vi "Get All LogMeasData from Q.vi"(8 "error in (no error)":errorcluster) -> (0 "error out":errorcluster, 1 "MeasData[] out":T1[](array[typedef]), 2 "NumElements":i32, 3 "orData out":T4)   [LabVIEW 2019]
doc: "Developed by Kevin Thompson\nThompson Engineering, LLC\nkevin@thompsonengineering.net"
uses:
  TD MeasData--cluster.ctl
  TD MeasData QRef.ctl
  GBL DataQ Ref.vi
  DataTypes/InverterData--cluster.ctl
  DataTypes/InverterPhaseData--cluster.ctl
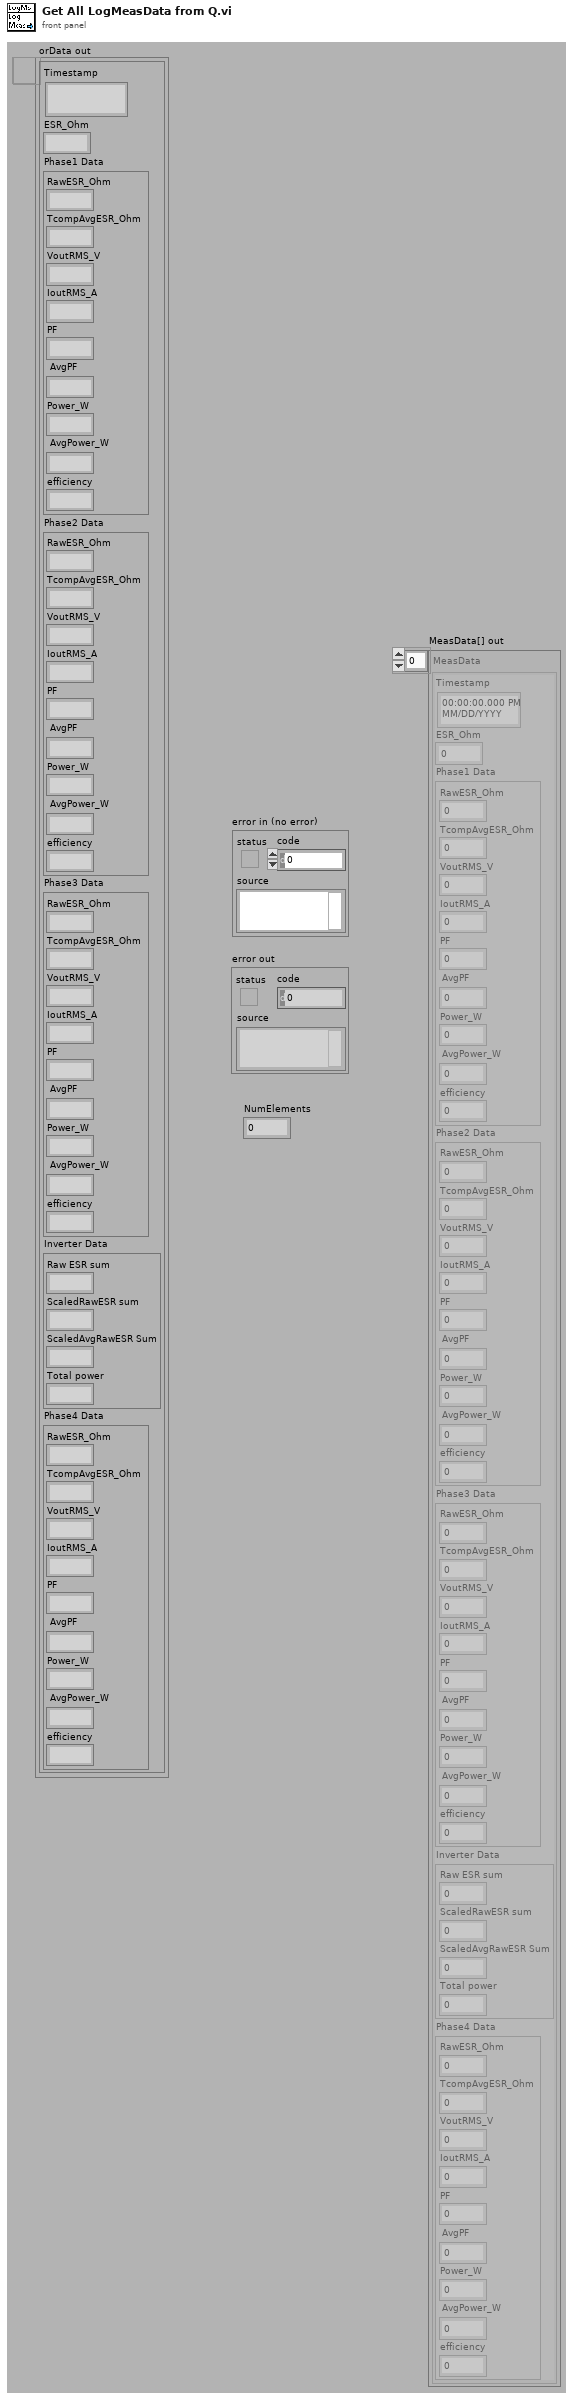
[diagram p1: front panel]
types:
  T1 = typedef "TD MeasData--cluster.ctl" = cluster{"Timestamp":timestamp, "ESR_Ohm":dbl, "Phase1 Data":T2, "Phase2 Data":T2, "Phase3 Data":T2, "Inverter Data":T3, "Phase4 Data":T2}
  T2 = typedef "InverterPhaseData--cluster.ctl" = cluster{"RawESR_Ohm":dbl, "TcompAvgESR_Ohm":dbl, "VoutRMS_V":dbl, "IoutRMS_A":dbl, "PF":dbl, "AvgPF":dbl, "Power_W":dbl, "AvgPower_W":dbl, "efficiency":dbl}
  T3 = typedef "InverterData--cluster.ctl" = cluster{"Raw ESR sum":dbl, "ScaledRawESR sum":dbl, "ScaledAvgRawESR Sum":dbl, "Total power":dbl}
  T4 = typedef "TD MeasData QRef.ctl" = refnum<queue>
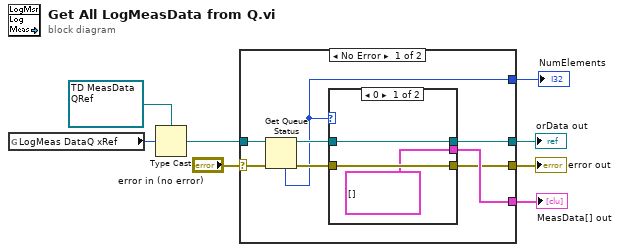
[diagram p0: block diagram]
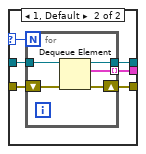
[diagram p2: hidden frame]
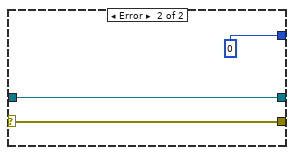
[diagram p3: hidden frame]
diagram:
  n1 = global read "GBL DataQ Ref.vi" "LogMeas DataQ xRef"() -> (w1:u32)
  n2 = Type Cast(type=T4 refnum ("orData out"), x=w1) -> (*(type *) &x=w5:T4)
  n3 = case shown="No Error" "error in (no error)" {
    selector: "error in (no error)" -> [w16 w32]
    tunnel: w5 -> [w15 w33]
    tunnel: [w10 w32] -> w8
    tunnel: [w14 w33] -> w7
    tunnel: [w11 _] -> w4
    tunnel: [w9 0 ("# elements in queue")] -> w3
    frame No Error {
      n4 = Get Queue Status(queue=w15, error in (no error)=w16) -> (queue out=w13:T4, error out=w12:errorcluster, # elements in queue=w9:i32)  [unwired: 1 in, 5 out]
      n5 = case shown="0" w9 {
        selector: w9 -> [_ w20]
        tunnel: [w19 w25] -> w14
        tunnel: w13 -> [w19 w24]
        tunnel: w12 -> [w18 w23]
        tunnel: [T1[] [] ("MeasData[] out") w22] -> w11
        tunnel: [w18 w21] -> w10
        frame 0 {
        }
        frame 1, Default {
          n6 = for {
            N: w20 -> [_]
            tunnel: [w30] -> w22 mode=indexing
            tunnel: [w29] -> w25
            tunnel: w24 -> [w28]
            shift-right: [w27] -> w21
            shift-left: w23 -> [w26]
            n7 = Dequeue Element(queue=w28, error in (no error)=w26) -> (queue out=w29:T4, element=w30:T1, error out=w27:errorcluster)  [unwired: 1 in, 1 out]
          }
        }
      }
    }
    frame Error {
    }
  }
  "orData out" <- w7
  "error out" <- w8
  "MeasData[] out" <- w4
  "NumElements" <- w3
